vi "Add Response (Result).vi"(5 "id value":string, 7 "jsonrpc":string, 8 "error in (no error)":errorcluster, 10 "JSON in":refnum<class "JSON Null.lvclass">, 11 "Server in":refnum<class "JSONRPC Server.lvclass">) -> (0 "error out":errorcluster, 1 "response string":string, 3 "Server out":refnum<class "JSONRPC Server.lvclass">)   [LabVIEW 2015, in "JSONRPC Server.lvclass"]
uses:
  JSONRPC Server.lvclass
  <vilib>/National Instruments/JSON Support for LabVIEW/JSON Data Classes/JSON Datatype/JSON Null.lvclass
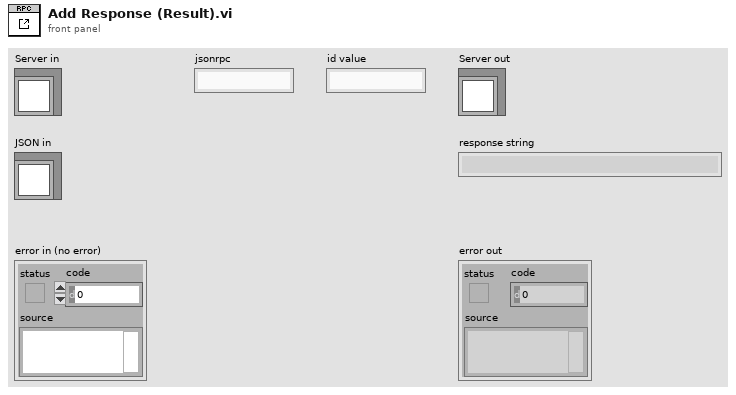
[diagram p1: front panel]
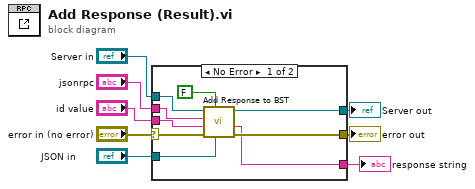
[diagram p0: block diagram]
diagram:
  n1 = case shown="No Error" "error in (no error)" {
    selector: "error in (no error)" -> [w13 w19]
    tunnel: [w14 w19] -> w6
    tunnel: [w16 w18] -> w5
    tunnel: "Server in" -> [w17 w18]
    tunnel: "jsonrpc" -> [w12 _]
    tunnel: "id value" -> [w11 _]
    tunnel: "JSON in" -> [w10 _]
    tunnel: [w9 _] -> w1
    frame No Error {
      n2 = call "Add Response to BST.vi"("JSON in"=w10, "error"=FALSE, "error in (no error)"=w13, "id value"=w11, "jsonrpc"=w12, "Server in"=w17) -> ("error out"=w14:errorcluster, "response string"=w9:string, "Server out"=w16:refnum<class "JSONRPC Server.lvclass">)  [unwired: 2 in, 1 out]
    }
    frame Error {
    }
  }
  "error out" <- w6
  "Server out" <- w5
  "response string" <- w1
